vi "Generic - AO1.vi"(0 "VISA session":refnum<visa-resource-name>="MW100", 2 "Semiphore":T1, 5 "Channel_Enum":T2=1 items=["4-20_OUT", "Pres_HI1", "Pres_HI2", "Pres_LOW", "Pres_PIN", "HEATER_TOP", "HEATER_BOT", "T_Shell", "FLOWMETER", "WATT_SENSE", "WH_TICK", "Tc_1", "Tc_2", "Tc_3", "Tc_4", "Tc_5", "Tc_6", "Tc_down", "T_Shell_2", "T_Shell_3", "T_Shell_4", "RTD_IN", "RTD_OUT", "RTD_AMB", "INTF_TEMPFLO", "INTF_READY", "INTF_START", "INTF_STOP", "DRM_LOW", "DRM_HIGH", "PWR_MAIN", "VLV_DUMP", "VLV_OUT", "VLV_IN", "WATT_HOURS", "FLOW(SAMPLE)", "GALLONS", "FLOW(GPM)", "FLOW_CALC_GAIN", "FLOW_CALC_OFFSET", "FLOW_CALC_THRESHOLD", "VLV_DUMP_2", "VLV_OUT_2", "VLV_IN_2", "VLV_DUMP_3", "VLV_OUT_3", "VLV_IN_3", "VLV_DUMP_4", "VLV_OUT_4", "VLV_IN_4", "CHAN_34", "CHAN_35", "CHAN_36"], 7 "Output Value (0)":i32, 11 "Error In":errorcluster) -> (4 "dup VISA session":refnum<visa-resource-name>, 15 "error out":errorcluster)   [LabVIEW 2012]
uses:
  ChannelSettings.ctl
panel:
  in  "Retries Allowed":i32=3
  in  "milliseconds to wait":u32=10
  out "Local?":bool
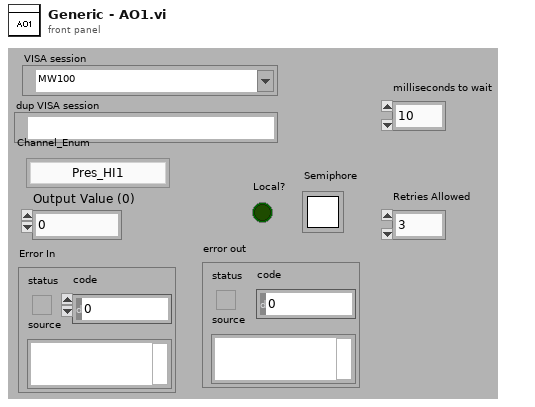
[diagram p1: front panel]
types:
  T1 = typedef "Semaphore RefNum" = refnum<k1>
  T2 = typedef "ChannelSettings.ctl" = u32
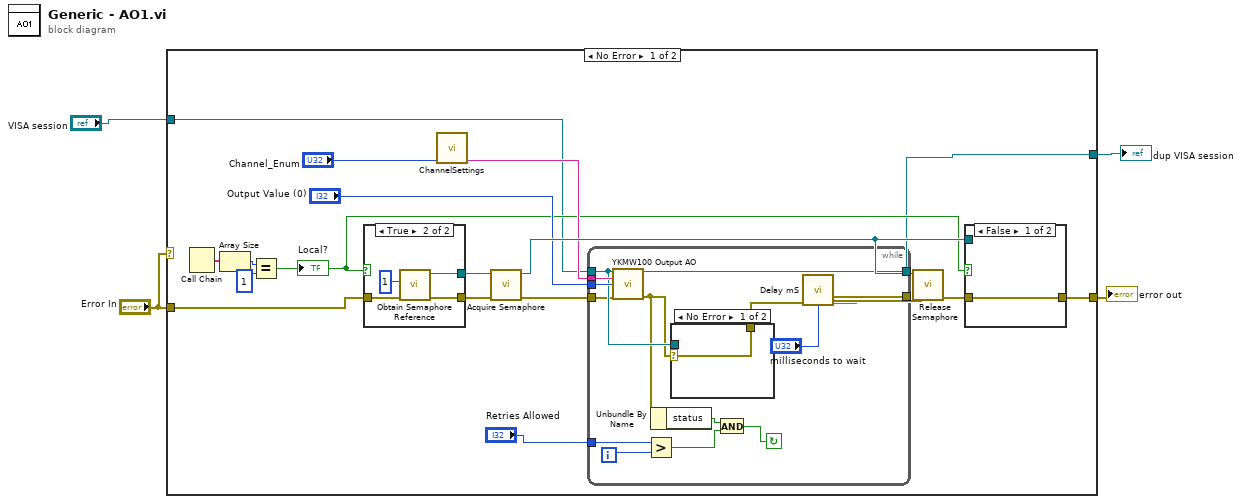
[diagram p0: block diagram]
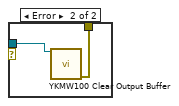
[diagram p2: hidden frame]
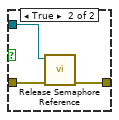
[diagram p3: hidden frame]
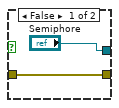
[diagram p4: hidden frame]
diagram:
  n1 = case shown="No Error" "Error In" {
    tunnel: "Error In" -> [w20 w50]
    tunnel: [w17 w50] -> w4
    tunnel: "VISA session" -> [w7 w51]
    tunnel: [w8 w51] -> w1
    frame No Error {
      n2 = Call Chain() -> (call chain=w10:string[])
      n3 = Array Size(array=w10) -> (size(s)=w11:i32)
      n4 = Equal?(x=w11, y=1) -> (x = y?=w9:bool)
      "Local?" <- w9
      n5 = case shown="True" w9 {
        tunnel: ["Semiphore" w48] -> w21
        tunnel: w20 -> [w45 w47]
        tunnel: [w45 w46] -> w19
        frame False {
        }
        frame True {
          n6 = call <vilib>:"Obtain Semaphore Reference.vi"("error in (no error)"=w47, "size (1)"=1) -> ("error out"=w46:errorcluster, "semaphore"=w48:T1)  [unwired: 3 in, 1 out]
        }
      }
      n7 = call "ChannelSettings.vi"("Channel_Enum"="Channel_Enum") -> ("Channel String"=w15:string)  [unwired: 10 in]
      n8 = call <vilib>:"Acquire Semaphore.vi"("error in (no error)"=w19, "semaphore"=w21) -> ("error out"=w13:errorcluster, "semaphore out"=w16:T1)  [unwired: 3 in, 1 out]
      n9 = while {
        tunnel: w15 -> [w36]
        tunnel: "Output Value (0)" -> [w35]
        tunnel: w13 -> [w28]
        tunnel: [w34] -> w8
        tunnel: [w29] -> w6
        tunnel: w7 -> [w33]
        tunnel: "Retries Allowed" -> [w24]
        i -> [w26]
        stop <- w32 continue-if-true
        n10 = call "YKMW100 Output AO.vi"("VISA session"=w33, "Channel String (001)"=w36, "Output Value (0)"=w35, "error in (no error)"=w28) -> ("dup VISA session"=w34:refnum<visa-resource-name>, "error out"=w27:errorcluster)  [unwired: 10 in]
        n11 = Greater?(x=w24, y=w26) -> (0:w25:bool)
        n12 = Unbundle By Name(w27) -> ("status"=w31:bool)
        n13 = case shown="No Error" w27 {
          selector: w27 -> [w37 _]
          tunnel: w33 -> [_ w39]
          tunnel: [w37 w38] -> w23
          frame No Error {
          }
          frame Error {
            n14 = call "YKMW100 Clear Output Buffer.vi"("VISA session"=w39) -> ("error out"=w38:errorcluster)  [unwired: 13 in, 1 out]
          }
        }
        n15 = And(x=w31, y=w25) -> (x .and. y?=w32:bool)
        n16 = call "Delay mS.vi"("Error In"=w23, "milliseconds to wait"="milliseconds to wait") -> ("Error Out"=w29:errorcluster)  [unwired: 13 in]
      }
      n17 = call <vilib>:"Release Semaphore.vi"("error in (no error)"=w6, "semaphore"=w16) -> ("error out"=w18:errorcluster)  [unwired: 4 in, 1 out]
      n18 = case shown="False" w9 {
        tunnel: w18 -> [w40 w43]
        tunnel: [w40 w42] -> w17
        tunnel: w16 -> [_ w41]
        frame False {
        }
        frame True {
          n19 = call <vilib>:"Release Semaphore Reference.vi"("error in (no error)"=w43, "semaphore"=w41) -> ("error out"=w42:errorcluster)  [unwired: 8 in, 1 out]
        }
      }
    }
    frame Error {
    }
  }
  "error out" <- w4
  "dup VISA session" <- w1
